vi "FindLowestPhaseShift.vi"(10 "all rows":string[][](array[string])) -> (1 "to return":i32, 2 "lowest phase":dbl)   [LabVIEW 2019]
panel:
  out "last is empty?":bool
  out "checked array":string[](array[string])
  out "decimated array":string[](array[string])
  out "lowest phase ind":i32
  out "subarray":string[][](array[string])
  # "should be between 12 and 20"
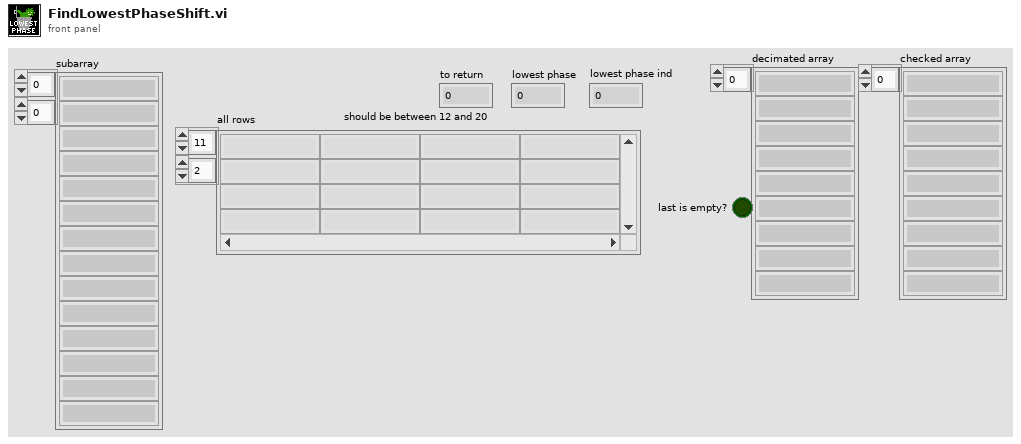
[diagram p1: front panel]
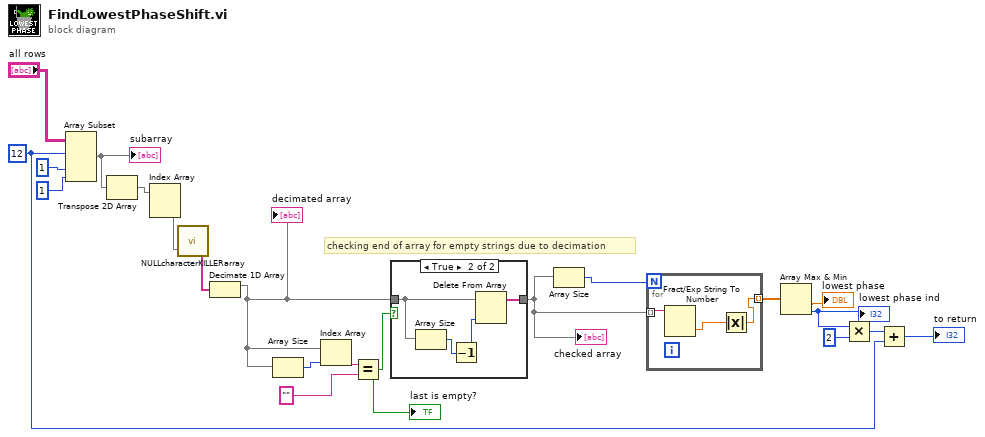
[diagram p0: block diagram]
diagram:
  w14 = 12 ("index")
  # "checking end of array for empty strings due to decimation"
  n1 = Array Subset(array="all rows", index (row)=w14, index (col)=1 ("index"), length (col)=1 ("length")) -> (w19:string[][])  [unwired: 1 in]
  "subarray" <- w19
  n2 = Transpose 2D Array(2D array=w19) -> (transposed array=w18:string[][])
  n3 = Index Array(array=w18) -> (element=w17:string[])  [unwired: 2 in]
  n4 = call "NULLcharacterKILLERarray.vi"("Input Array"=w17) -> ("Cleaned Array"=w16:string[])  [unwired: 1 in]
  n5 = Decimate 1D Array(w16) -> (w3:string[])  [unwired: 1 out]
  "decimated array" <- w3
  n6 = Array Size(array=w3) -> (size(s)=w9:i32)
  n7 = Index Array(array=w3, index=w9) -> (element=w8:string)
  n8 = Equal?(x=w8, y="") -> (x = y?=w7:bool)
  "last is empty?" <- w7
  n9 = case shown="True" w7 {
    tunnel: w3 -> [w22 w25]
    tunnel: [w22 w26] -> w5
    frame False {
    }
    frame True {
      n10 = Array Size(array=w25) -> (size(s)=w24:i32)
      n11 = Decrement(x=w24) -> (x-1=w23:i32)
      n12 = Delete From Array(array=w25, index=w23) -> (array with subset deleted=w26:string[])  [unwired: 1 in, 1 out]
    }
  }
  "checked array" <- w5
  n13 = Array Size(array=w5) -> (size(s)=w6:i32)
  n14 = for {
    N: w6 -> [_]
    tunnel: w5 -> [w29] mode=indexing
    tunnel: [w27] -> w4 mode=indexing
    n15 = Fract/Exp String To Number(string=w29) -> (number=w28:dbl)  [unwired: 3 in, 1 out]
    n16 = Absolute Value(x=w28) -> (abs(x)=w27:dbl)
  }
  n17 = Array Max & Min(array=w4) -> (min value=→"lowest phase":dbl, min index (indices)=w1:i32)  [unwired: 2 out]
  "lowest phase ind" <- w1
  n18 = Multiply(x=w1, y=2) -> (x*y=w12:i32)
  n19 = Add(x=w12, y=w14) -> (x+y=→"to return":i32)
